vi "专用-遍历扫描串口探头.vi"(8 "发现的探头[]-引用":refnum<vi>, 9 "扫描结果-引用":refnum<vi>, 10 "扫描进度-引用":refnum<vi>, 11 "扫描按钮-引用":refnum<vi>) -> ()   [LabVIEW 2017]
uses:
  06948e99-37de-4c6b-809c-0b83fd37c0e4.vi
panel:
  out "保存过得串口探头":u16[](array[numeric])
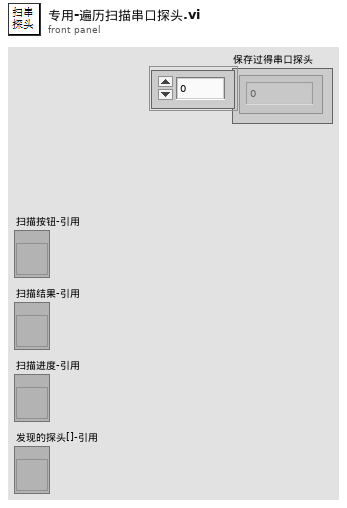
[diagram p1: front panel]
types:
  T1 = typedef "测量值读取.ctl" = cluster{"测量值":dbl, "CRC":bool, "接收指令":string}
  T2 = typedef "串口配置.ctl" = cluster{"COM口":refnum<visa-resource-name>, "波特率":enum16{"9600", "19200"}, "探头地址(U8)":u8}
  T3 = typedef "串口动作类型.ctl" = enum16{"读测量值", "设置报警值", "设置地址", "设置系数", "广播修改波特率", "关闭串口"}
  T4 = typedef "串口模块输入.ctl" = cluster{"串口动作类型":T3, "串口配置":T2, "数据输入":variant}
  T5 = typedef "探测器信息.ctl" = cluster{"网络地址":string, "名称":string, "备注":string, "累积剂量":dbl, "累积限值":dbl, "硬件剂量率限值":T6, "剂量率限值1":dbl, "剂量率限值2":dbl, "报警方式":T7}
  T6 = typedef "探头剂量率限值选择.ctl" = enum16{"一级限值", "二级限值"}
  T7 = typedef "报警方式选择.ctl" = enum16{"常报警", "自动静音", "手动静音"}
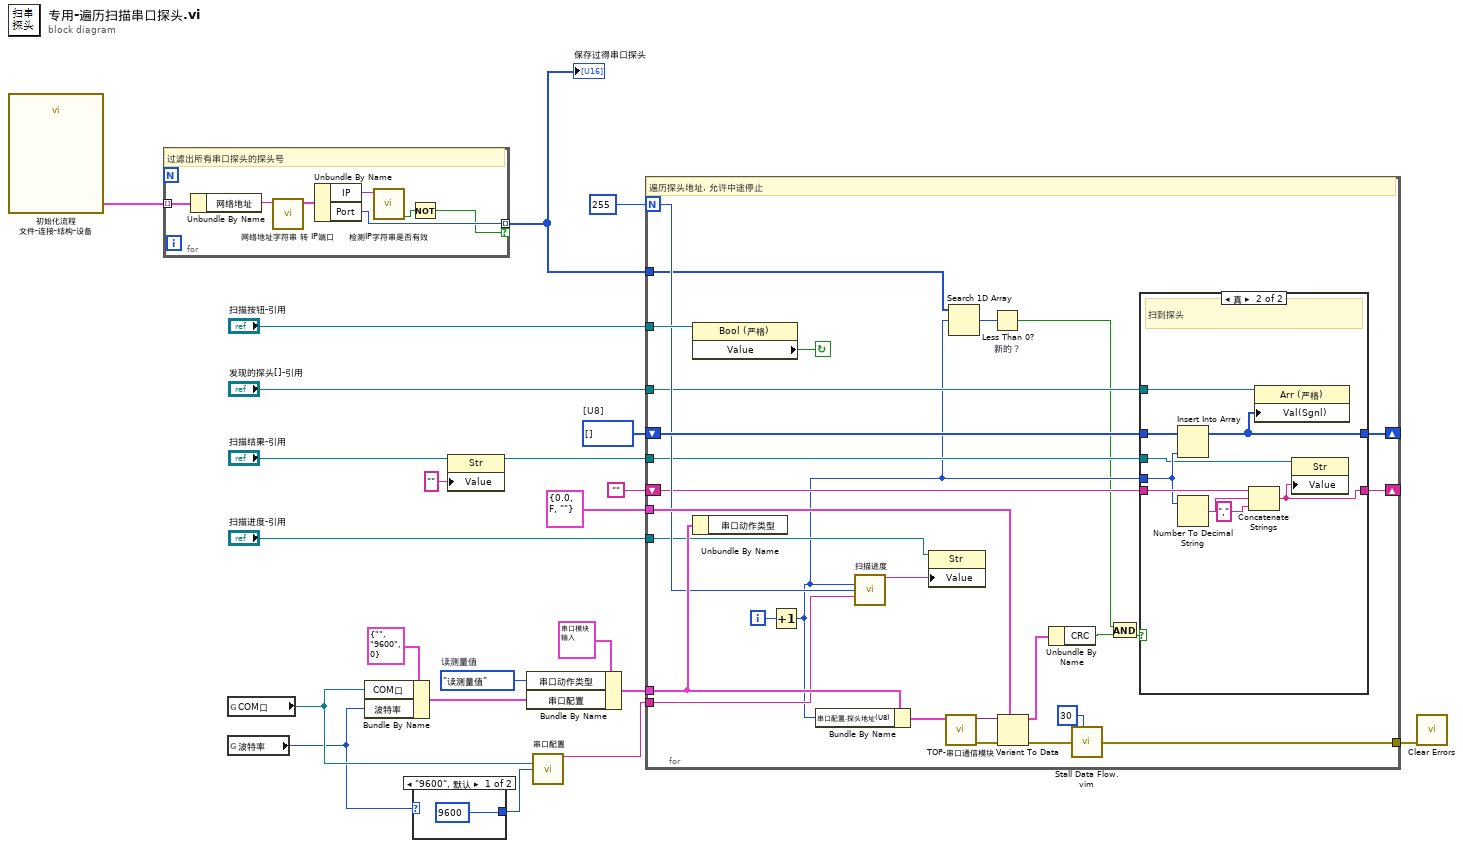
[diagram p0: block diagram]
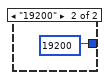
[diagram p2: hidden frame]
diagram:
  w13 = u8[] []  # [U8]
  w19 = 串口动作类型."读测量值"  # 读测量值
  n1 = call "初始化流程 文件-连接-结构-设备.vi"() -> ("探测器信息[]"=w4:T5[])  [unwired: 10 in, 1 out]
  n2 = for {
    tunnel: w4 -> [w29] mode=indexing
    tunnel: [w25] -> w3 mode=indexing if=w23
    # "过滤出所有串口探头的探头号"
    n3 = Unbundle By Name(w29) -> ("网络地址"=w27:string)
    n4 = call "网络地址字符串 转 IP端口.vi"("IP端口字符串"=w27) -> ("IP端口"=w28:cluster{"IP":string, "Port":u16})  [unwired: 10 in]
    n5 = Unbundle By Name(w28) -> ("IP"=w26:string, "Port"=w25:u16)
    n6 = call "检测IP字符串是否有效.vi"("IP地址"=w26) -> ("有效IP？"=w24:bool)  [unwired: 10 in]
    n7 = Not(x=w24) -> (.not. x?=w23:bool)
  }
  "保存过得串口探头" <- w3
  n8 = global read "全局变量-35点监测.vi" "COM口"() -> (w12:refnum<visa-resource-name>)
  n9 = global read "全局变量-35点监测.vi" "波特率"() -> (w6:enum16{"9600", "19200"})
  n10 = Bundle By Name(cluster=T2 {"COM口"="", "波特率"=enum."9600", "探头地址(U8)"=0} ("串口配置"), "COM口"=w12, "波特率"=w6) -> (w17:T2)
  n11 = case shown="\"9600\", 默认" w6 {
    tunnel: [9600 19200] -> w5
    frame "9600", Default {
    }
    frame "19200" {
    }
  }
  n12 = property class="Str"(reference="扫描结果-引用", "Value"="" ("值")) -> (reference out=w2:refnum<vi>)  [unwired: 1 in, 1 out]
  n13 = Bundle By Name(cluster=T4 {"串口动作类型"=enum."读测量值", "串口配置"={"COM口"="", "波特率"=enum."9600", "探头地址(U8)"=0}, "数据输入"=variant} ("串口模块输入"), "串口动作类型"=w19, "串口配置"=w17) -> (w16:T4)
  n14 = call "串口配置"("COM"=w12, "波特率"=w5) -> ("Result"=w11:string)  [unwired: 12 in, 1 out]
  n15 = for {
    N: u8 255 -> [w47]
    tunnel: "扫描按钮-引用" -> [w59]
    tunnel: w16 -> [w48]
    tunnel: T1 {"测量值"=0.0, "CRC"=FALSE, "接收指令"=""} ("测量值读取") -> [w54]
    tunnel: [w40] -> w14
    shift-right: [w37] -> _
    shift-left: w13 -> [w50]
    tunnel: w11 -> [w46]
    tunnel: "扫描进度-引用" -> [w45]
    shift-right: [w42] -> _
    shift-left: "" -> [w43]
    tunnel: w2 -> [w41]
    tunnel: "发现的探头[]-引用" -> [w38]
    tunnel: w3 -> [w36]
    i -> [w51]
    stop <- w58 continue-if-true
    # "遍历探头地址, 允许中途停止"
    n16 = property class="Bool (严格)"(reference=w59) -> ("Value"=w58:bool)  [unwired: 1 in, 2 out]
    n17 = Unbundle By Name(w48) -> ()  [unwired: 1 out]
    n18 = Increment(x=w51) -> (x+1=w35:i32)
    n19 = Bundle By Name(cluster=w48, "串口配置.探头地址(U8)"=w35) -> (w52:T4)
    n20 = call "扫描进度"("当前探头号"=w35, "总数"=w47, "串口配置"=w46) -> ("Result"=w44:string)  [unwired: 11 in, 1 out]
    n21 = property class="Str"(reference=w45, "Value"=w44) -> ()  [unwired: 1 in, 2 out]
    n22 = call "TOP-串口通信模块.vi"("串口模块输入"=w52) -> ("error out"=w57:errorcluster, "数据输出"=w55:variant)  [unwired: 9 in]
    n23 = Search 1D Array(1D array=w36, element=w35) -> (index of element=w34:i32)  [unwired: 1 in]
    n24 = Less Than 0? "新的？"(x=w34) -> (x < 0?=w32:bool)
    n25 = Variant To Data(error in=w57, type=w54, Variant=w55) -> (data=w56:T1, error out=w53:errorcluster)
    n26 = Unbundle By Name(w56) -> ("CRC"=w49:bool)
    n27 = call "Stall Data Flow.vim"("value in"=w53, "milliseconds to wait"=u32 30) -> ("value out"=w40:errorcluster)  [unwired: 1 out]
    n28 = And(x=w32, y=w49) -> (x .and. y?=w33:bool)
    n29 = case shown="真" w33 {
      tunnel: w50 -> [w61 w70]
      tunnel: w35 -> [_ w68]
      tunnel: [w61 w62] -> w37
      tunnel: w43 -> [w60 w69]
      tunnel: [w60 w65] -> w42
      tunnel: w41 -> [_ w64]
      tunnel: w38 -> [_ w63]
      frame False {
        # "没有探头"
      }
      frame True {
        # "扫到探头"
        n30 = Insert Into Array(array=w70, new element=w68) -> (w62:u8[])  [unwired: 1 in]
        n31 = Number To Decimal String(number=w68) -> (decimal integer string=w67:string)  [unwired: 1 in]
        n32 = Concatenate Strings(w69, w67, ",") -> (w65:string)
        n33 = property class="Arr (严格)"(reference=w63, "Val(Sgnl)"=w62) -> ()  [unwired: 1 in, 2 out]
        n34 = property class="Str"(reference=w64, "Value"=w65) -> ()  [unwired: 1 in, 2 out]
      }
    }
  }
  n35 = call <vilib>:"Clear Errors.vi"("error in (no error)"=w14) -> ()  [unwired: 5 in, 2 out]
